vi "showResults.vi"(0 "reference in":refnum<class "subject.lvclass">, 11 "error in (no error)":errorcluster) -> (3 "data":T1, 4 "reference out":refnum<class "subject.lvclass">, 6 "results_user_selection":T2, 8 "results_5l":T2, 10 "results_15percent":T2, 14 "supportData":T3, 15 "error out":errorcluster)   [LabVIEW 2015, in "subject.lvclass"]
uses:
  subject.lvclass
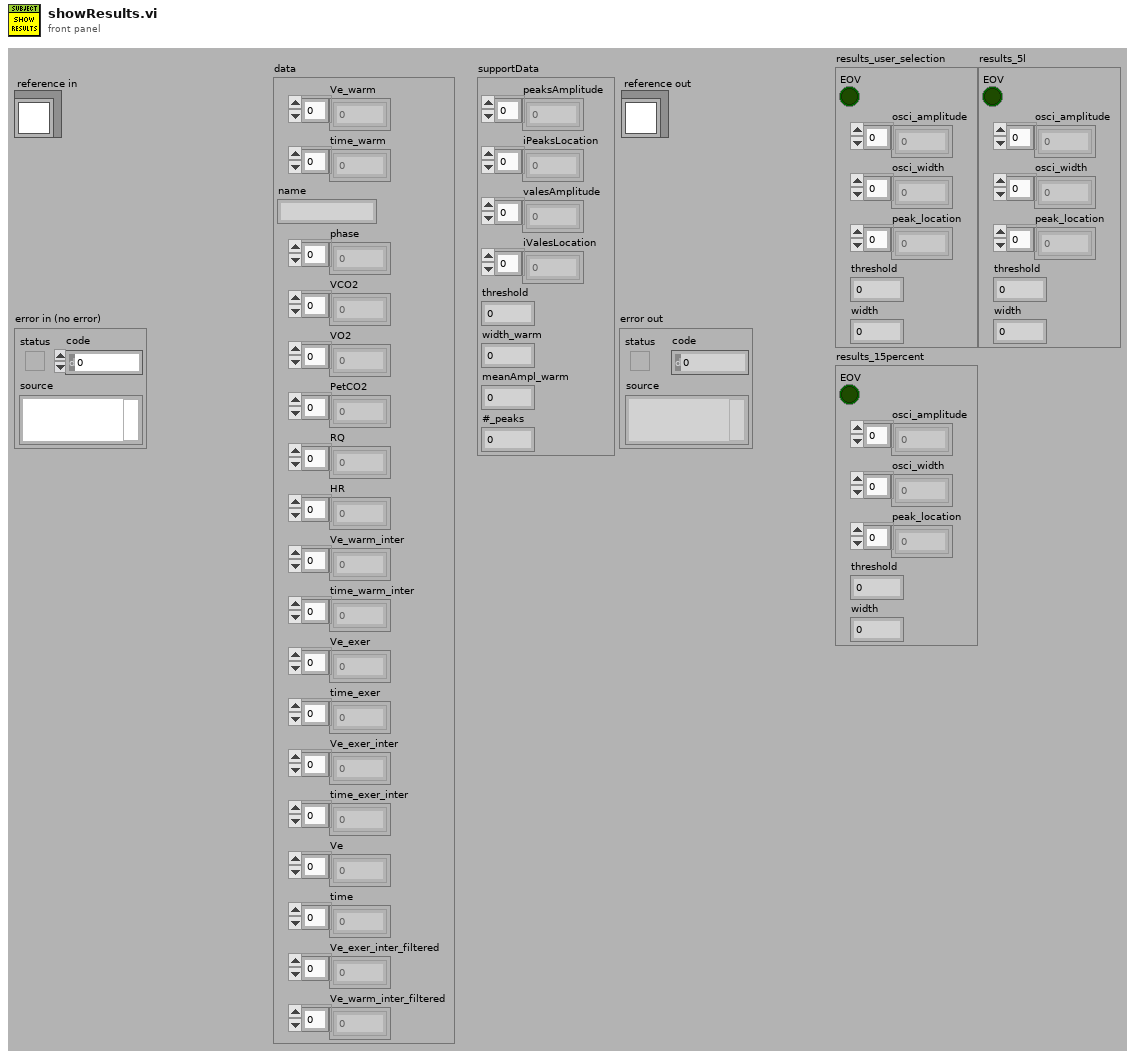
[diagram p1: front panel]
types:
  T1 = cluster{"Ve_warm":dbl[], "time_warm":dbl[], "name":string, "phase":dbl[], "VCO2":dbl[], "VO2":dbl[], "PetCO2":dbl[], "RQ":dbl[], "HR":dbl[], "Ve_warm_inter":dbl[], "time_warm_inter":dbl[], "Ve_exer":dbl[], "time_exer":dbl[], "Ve_exer_inter":dbl[], "time_exer_inter":dbl[], "Ve":dbl[], "time":dbl[], "Ve_exer_inter_filtered":dbl[], "Ve_warm_inter_filtered":dbl[]}
  T2 = cluster{"EOV":bool, "osci_amplitude":dbl[], "osci_width":dbl[], "peak_location":dbl[], "threshold":dbl, "width":i32}
  T3 = cluster{"peaksAmplitude":dbl[], "iPeaksLocation":dbl[], "valesAmplitude":dbl[], "iValesLocation":dbl[], "threshold":dbl, "width_warm":i32, "meanAmpl_warm":i32, "#_peaks":i32}
  T4 = typedef "subject.lvclass/ObjectAttributesRef.ctl" = refnum<data-value>
  T5 = typedef "subject.lvclass/ObjectAttributes.ctl" = cluster{"MyAttribute":dbl, "data":cluster{"Ve_warm":dbl[], "time_warm":dbl[], "name":string, "phase":dbl[], "VCO2":dbl[], "VO2":dbl[], "PetCO2":dbl[], "RQ":dbl[], "HR":dbl[], "Ve_warm_inter":dbl[], "time_warm_inter":dbl[], "Ve_exer":dbl[], "time_exer":dbl[], "Ve_exer_inter":dbl[], "time_exer_inter":dbl[], "Ve":dbl[], "time":dbl[], "Ve_exer_inter_filtered":dbl[], "Ve_warm_inter_filtered":dbl[]}, "results_5l":cluster{"EOV":bool, "osci_amplitude":dbl[], "osci_width":dbl[], "peak_location":dbl[], "threshold":dbl, "width":i32}, "results_15percent":cluster{"EOV":bool, "osci_amplitude":dbl[], "osci_width":dbl[], "peak_location":dbl[], "threshold":dbl, "width":i32}, "supportData":cluster{"peaksAmplitude":dbl[], "iPeaksLocation":dbl[], "valesAmplitude":dbl[], "iValesLocation":dbl[], "threshold":dbl, "meanAmpl_warm":i32, "#_peaks":i32, "width":i32}, "results_user_selection":cluster{"EOV":bool, "osci_amplitude":dbl[], "osci_width":dbl[], "peak_location":dbl[], "threshold":dbl, "width":i32}, "results_warm_up":cluster{"EOV":bool, "osci_amplitude":dbl[], "osci_width":dbl[], "peak_location":dbl[], "threshold":dbl, "width":i32}}
  T6 = cluster{"peaksAmplitude":dbl[], "iPeaksLocation":dbl[], "valesAmplitude":dbl[], "iValesLocation":dbl[], "threshold":dbl, "meanAmpl_warm":i32, "#_peaks":i32, "width":i32}
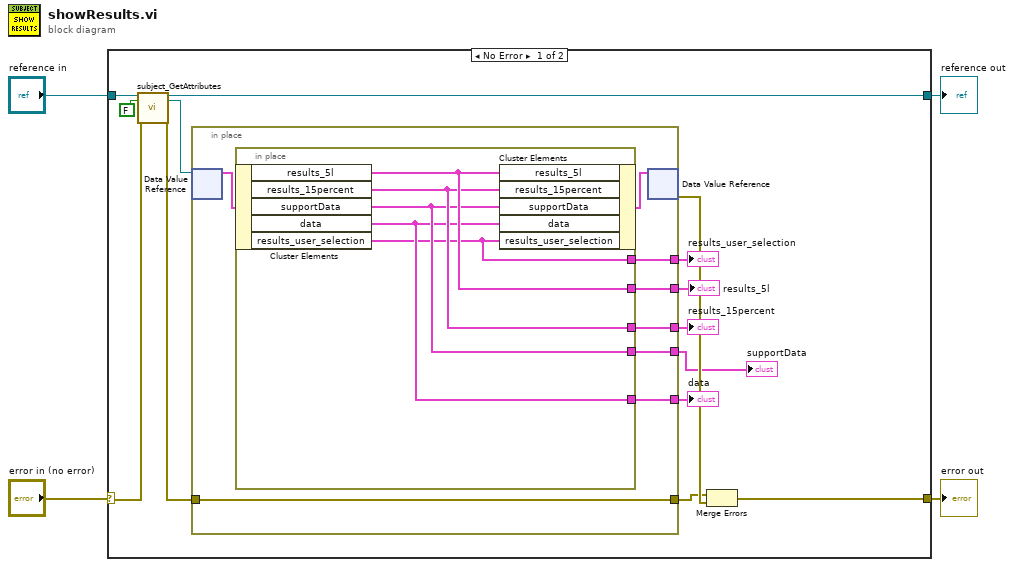
[diagram p0: block diagram]
diagram:
  n1 = case shown="No Error" "error in (no error)" {
    selector: "error in (no error)" -> [w13 w33]
    tunnel: [w18 w33] -> w3
    tunnel: [w11 w32] -> w1
    tunnel: "reference in" -> [w15 w32]
    frame No Error {
      n2 = call "subject_GetAttributes.vi"("reference in"=w15, "return data? (T)"=FALSE, "error in (no error)"=w13) -> ("reference out"=w11:refnum<class "subject.lvclass">, "attributes ref"=w10:T4, "error out"=w12:errorcluster)  [unwired: 13 in, 1 out]
      n3 = in-place {
        in-place-border: w12 -> [w24]
        in-place-border: [w24] -> w16
        in-place-border: [w23] -> w7
        in-place-border: [w22] -> w6
        in-place-border: [w21] -> w9
        in-place-border: [w20] -> w5
        in-place-border: [w19] -> w8
        n4 = in-place-dvr #1(w10) -> (w25:T5)  [unwired: 1 out]
        n5 = in-place {
          in-place-border: [w31] -> w23
          in-place-border: [w30] -> w22
          in-place-border: [w29] -> w21
          in-place-border: [w28] -> w20
          in-place-border: [w27] -> w19
          n6 = in-place-cluster #2(w25) -> ("results_5l"=w31:T2, "results_15percent"=w30:T2, "supportData"=w29:T6, "data"=w28:T1, "results_user_selection"=w27:T2)
          n7 = in-place-cluster #2("results_5l"=w31, "results_15percent"=w30, "supportData"=w29, "data"=w28, "results_user_selection"=w27) -> (w26:T5)
        }
        n8 = in-place-dvr #1(w26) -> (w17:errorcluster)  [unwired: 1 out]
      }
      "supportData" <- w9
      "results_user_selection" <- w8
      "results_5l" <- w7
      "results_15percent" <- w6
      "data" <- w5
      n9 = Merge Errors(w16, w17) -> (w18:errorcluster)
    }
    frame Error {
    }
  }
  "error out" <- w3
  "reference out" <- w1
